vi "LSX Set Encoder Position.vi"(8 "error in (no error)":errorcluster, 10 "bValue":i32, 11 "lLSID":i32) -> (0 "error out":errorcluster, 3 "function return":i32)   [LabVIEW 2018, in "Tango.lvlib"]
doc: "TANGOAPI int TANGOCALL LSX_SetEncoderPosition (int lLSID, BOOL bValue);"
uses:
  Tango.lvlib
  SubVIs/Tango_DLL.dll
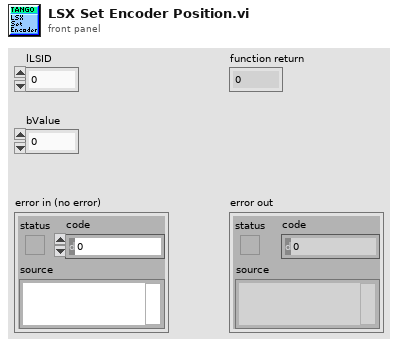
[diagram p1: front panel]
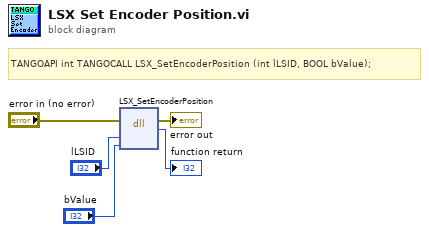
[diagram p0: block diagram]
diagram:
  # "TANGOAPI int TANGOCALL LSX_SetEncoderPosition (int lLSID, BOOL bValue);"
  n1 = dll-call lib="C:/Users/Familie/Documents/LabviewIX81/lib/TANGO Stage/SubVIs/Tango_DLL.*" fn="LSX_SetEncoderPosition"(error in="error in (no error)", "lLSID"="lLSID", "bValue"="bValue") -> (error out=→"error out":errorcluster, →"function return":i32)  [unwired: 4 in, 1 out]
